vi "WriteEEPROM.vi"(4 "Write Data to EEPROM":bool, 5 "Query":string, 6 "Data":dbl[](array[numeric]), 7 "Command":string, 8 "error in":errorcluster, 10 "Skip":bool, 11 "VISA resource name":refnum<visa-resource-name>) -> (0 "error out":errorcluster, 1 "Checked Data":dbl[](array[numeric]), 2 "Write Successful":bool, 3 "VISA resource name out":refnum<visa-resource-name>)   [LabVIEW 2010]
uses:
  Instance           1 19Saved   WriteEEPROM .vi
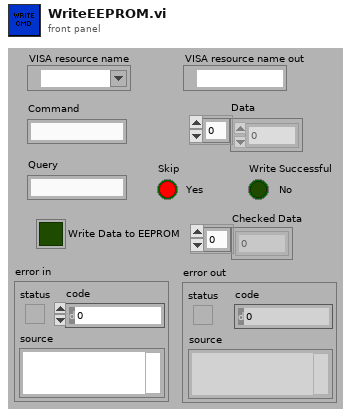
[diagram p1: front panel]
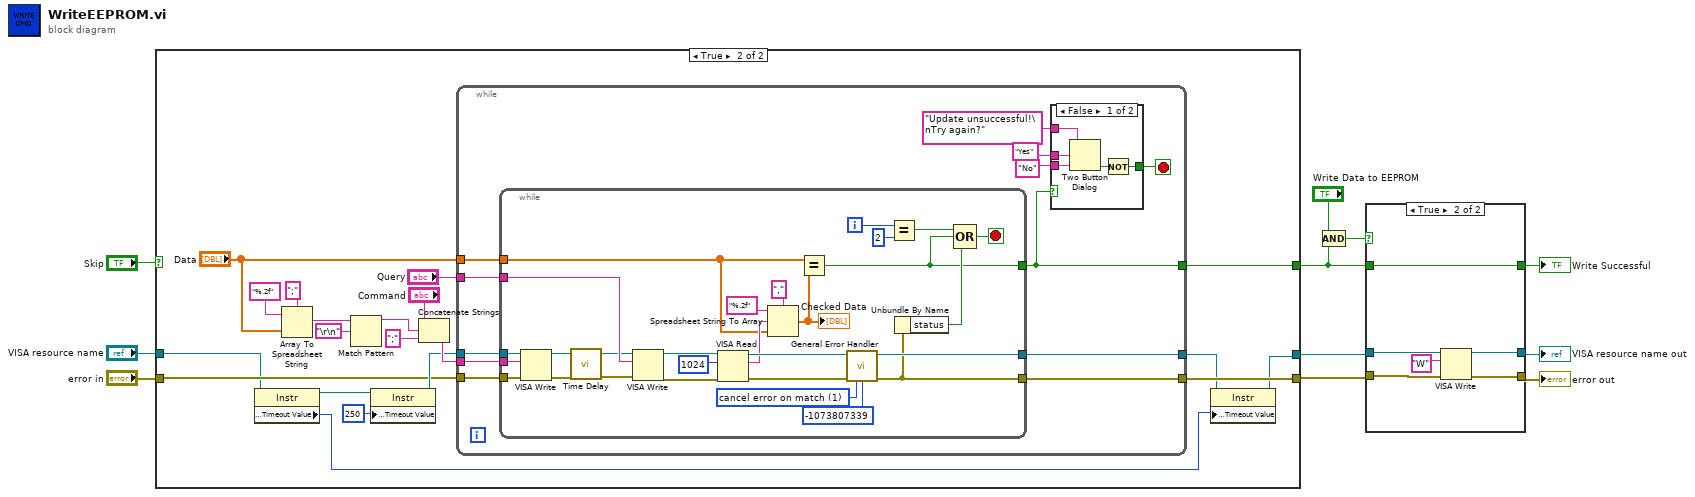
[diagram p0: block diagram]
diagram:
  n1 = case shown="True" "Skip" {
    selector: "Skip" -> [w14 _]
    tunnel: [w14 w33] -> w1
    tunnel: [w12 w17] -> w11
    tunnel: [w13 w26] -> w10
    tunnel: "error in" -> [w13 w21]
    tunnel: "VISA resource name" -> [w12 w20]
    frame False {
    }
    frame True {
      n2 = property class="Instr"(reference=w20) -> (reference out=w19:refnum<visa-resource-name>, "General Settings:Timeout Value"=w16:u32)  [unwired: 1 in, 1 out]
      n3 = Array To Spreadsheet String(delimiter (Tab)=";", array="Data", 3:"%.2f" ("format string")) -> (spreadsheet string=w28:string)
      n4 = Match Pattern(string=w28, regular expression="\r\n") -> (before substring=w15:string)  [unwired: 4 out]
      n5 = property class="Instr"(reference=w19, "General Settings:Timeout Value"=u32 250) -> (reference out=w22:refnum<visa-resource-name>)  [unwired: 1 in, 1 out]
      n6 = Concatenate Strings("Command", w15, ";" ("string")) -> (w30:string)
      n7 = while {
        tunnel: [w36] -> w33
        tunnel: w30 -> [w46]
        tunnel: [w45] -> w26
        tunnel: "Query" -> [w44]
        tunnel: "Data" -> [w43]
        tunnel: w22 -> [w42]
        tunnel: w21 -> [w41]
        tunnel: [w40] -> w18
        stop <- w35 stop-if-true
        n8 = while {
          tunnel: w42 -> [w78]
          tunnel: w46 -> [w77]
          tunnel: [w54] -> w36
          tunnel: [w75] -> w40
          tunnel: w41 -> [w68]
          tunnel: [w60] -> w45
          tunnel: w44 -> [w66]
          tunnel: w43 -> [w62]
          i -> [w74]
          stop <- w71 stop-if-true
          w58 = 1 items=["no exception", "cancel error on match", "set error on match"] ("[exception action] (none:0)")
          n9 = VISA Write(VISA resource name=w78, write buffer=w77, error in (no error)=w68) -> (VISA resource name out=w53:refnum<visa-resource-name>, error out=w56:errorcluster)  [unwired: 1 out]
          n10 = call "Time Delay"("error in (no error)"=w56) -> ("error out"=w55:errorcluster)  [unwired: 1 in, 9 out]
          n11 = VISA Write(VISA resource name=w53, write buffer=w66, error in (no error)=w55) -> (VISA resource name out=w70:refnum<visa-resource-name>, error out=w67:errorcluster)  [unwired: 1 out]
          n12 = VISA Read(VISA resource name=w70, byte count=u32 1024, error in (no error)=w67) -> (VISA resource name out=w75:refnum<visa-resource-name>, read buffer=w63:string, error out=w59:errorcluster)  [unwired: 1 out]
          n13 = Spreadsheet String To Array(delimiter (Tab)=",", format string="%.2f", spreadsheet string=w63, array type (2D Dbl)=w62) -> (array=w61:dbl[])
          "Checked Data" <- w61
          n14 = Equal?(x=w62, y=w61) -> (x = y?=w54:bool)
          n15 = call <vilib>:"General Error Handler.vi"("error in (no error)"=w59, "[exception action] (none:0)"=w58, "[exception code]"=-1073807339) -> ("error out"=w60:errorcluster)  [unwired: 1 in, 11 out]
          n16 = Equal?(x=w74, y=2) -> (x = y?=w72:bool)
          n17 = Unbundle By Name(w60) -> ("status"=w69:bool)
          n18 = Compound Arithmetic op=OR(w72, w54, w69) -> (w71:bool)
        }
        n19 = case shown="False" w36 {
          selector: w36 -> [_ w52]
          tunnel: [w47 w52] -> w35
          tunnel: "Update unsuccessful!\nTry again?" -> [w50 _]
          tunnel: "Yes" -> [w49 _]
          tunnel: "No" -> [w48 _]
          frame False {
            n20 = Two Button Dialog(message=w50, 1:w48, 2:w49) -> (T button?=w51:bool)
            n21 = Not(x=w51) -> (.not. x?=w47:bool)
          }
          frame True {
          }
        }
      }
      n22 = property class="Instr"(reference=w18, "General Settings:Timeout Value"=w16) -> (reference out=w17:refnum<visa-resource-name>)  [unwired: 1 in, 1 out]
    }
  }
  n23 = Compound Arithmetic op=AND("Write Data to EEPROM", w1) -> (w3:bool)
  n24 = case shown="True" w3 {
    tunnel: w11 -> [w80 w87]
    tunnel: w10 -> [w81 w83]
    tunnel: [w81 w82] -> w9
    tunnel: [w80 w85] -> w8
    tunnel: [w79 w84] -> w7
    tunnel: w1 -> [w79 w84]
    frame False {
    }
    frame True {
      n25 = VISA Write(VISA resource name=w87, write buffer="W", error in (no error)=w83) -> (VISA resource name out=w85:refnum<visa-resource-name>, error out=w82:errorcluster)  [unwired: 1 out]
    }
  }
  "Write Successful" <- w7
  "error out" <- w9
  "VISA resource name out" <- w8
